vi "Error Global.vi"() -> ()   [LabVIEW 2025, in "I2C Bus Monitor.lvclass"]
uses:
  I2C Bus Monitor.lvclass
panel:
  out "-8052":string="\nEmpty Resource Name\n\nPossible Reason(s):\nThe plugin was unable to find a supported device on this system.\n\nSupported Models:\n%s"
  out "-8051":string="\nEmpty or Invalid Bitfile Path\n\nPossible Reason(s):\nThe plugin was unable to find a bitfile for the specified device in the following directory:\n\n\"%s\""
  out "-8050":string="\nUnable to Open FPGA Session\n\nPossible Reason(s):\nThere's another session using the same FPGA resource with a different bitfile.\n\nIf you want to use this plugin in parallel to another session using the same FPGA resource, then you must use one of the bitfiles that corresponds to your device model in this directory:\n\n\"%s\"\n\nFor example, for this session, the plugin has used the following bitfile:\n\n\"%s\""
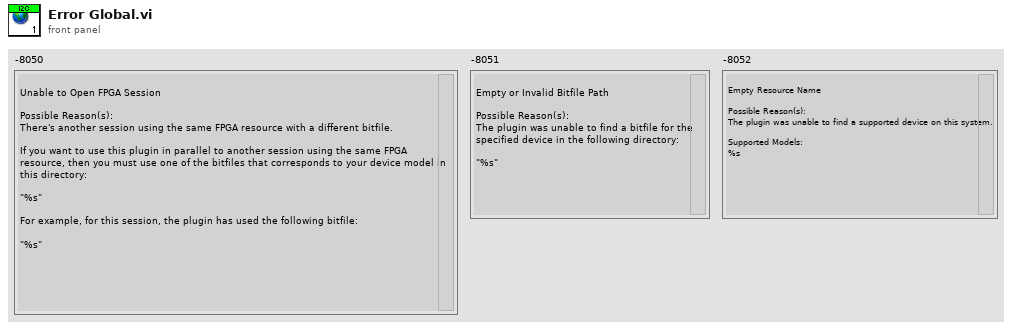
[diagram p1: front panel]
diagram:
